vi "isLeapYear (Poly).vi"   [LabVIEW 2017]
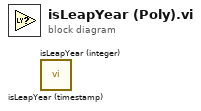
[diagram p0: block diagram]
diagram:
  n1 = call "isLeapYear (timestamp).vi"() -> ()  [unwired: 9 in, 1 out]
  n2 = call "isLeapYear (integer).vi"() -> ()  [unwired: 9 in, 1 out]
